vi "Save2DArrayWithColumnNames.vi"(7 "format (%6e)":string="%6e", 8 "error in (no error)":errorcluster, 9 "2D data":dbl[][](array[numeric]), 10 "Column name array":string[](array[string]), 11 "path in":path) -> (0 "error out":errorcluster, 3 "path out":path)   [LabVIEW 2020, in "Initialization.lvlib" / "FileManagement.lvlib"]
uses:
  FileManagement.lvlib
  <vilib>/Utility/error.llb/DialogType.ctl
  <vilib>/Utility/file.llb/Write To Spreadsheet File (DBL).vi
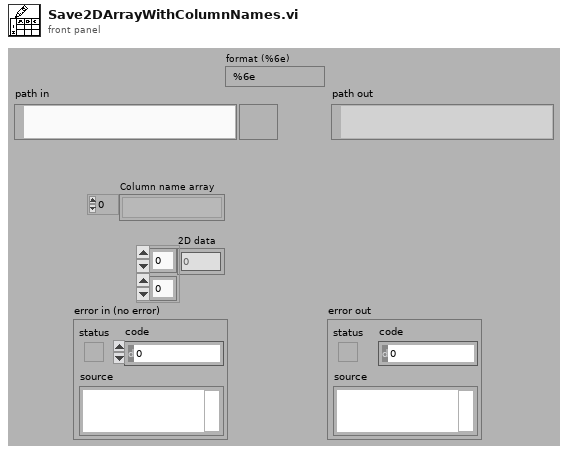
[diagram p1: front panel]
types:
  T1 = enum16{"open", "replace", "create", "open or create", "replace or create", "replace or create with confirmation"}
  T2 = typedef "DialogType.ctl" = u16
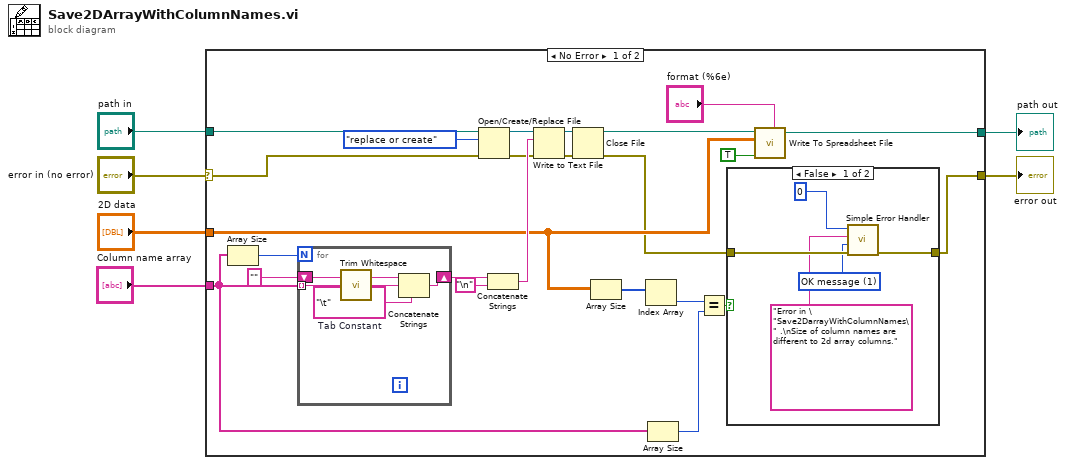
[diagram p0: block diagram]
diagram:
  n1 = case shown="No Error" "error in (no error)" {
    selector: "error in (no error)" -> [w17 w43]
    tunnel: "path in" -> [w16 w42]
    tunnel: "2D data" -> [w15 _]
    tunnel: [w29 w42] -> w5
    tunnel: "Column name array" -> [w14 _]
    tunnel: [w8 w43] -> w4
    frame No Error {
      n2 = Array Size(array=w14) -> (size(s)=w28:i32)
      n3 = for {
        N: w28 -> [_]
        tunnel: w14 -> [w38] mode=indexing
        shift-right: [w41] -> w25
        shift-left: "" -> [w39]
        w40 = "\t"  # Tab Constant
        n4 = call <vilib>:"Trim Whitespace.vi"("string"=w38) -> ("trimmed string"=w37:string)  [unwired: 1 in]
        n5 = Concatenate Strings(w39, w37, w40) -> (w41:string)
      }
      n6 = Open/Create/Replace File(file path (use dialog)=w16, error in=w17, operation (0:open)=T1."replace or create" ("操作(0:open)")) -> (refnum out=w22:refnum<file>, error out=w20:errorcluster)  [unwired: 3 in, 1 out]
      n7 = Concatenate Strings(w25, "\n") -> (w26:string)
      n8 = Write to Text File(file (use dialog)=w22, text=w26, error in=w20) -> (refnum out=w21:refnum<file>, error out=w19:errorcluster)  [unwired: 1 in, 1 out]
      n9 = Close File(refnum=w21, error in=w19) -> (path=w30:path, error out=w9:errorcluster)
      n10 = Array Size(array=w15) -> (size(s)=w13:i32[])
      n11 = Index Array(array=w13) -> (element=w12:i32)  [unwired: 1 in]
      n12 = Array Size(array=w14) -> (size(s)=w11:i32)
      n13 = Equal?(x=w12, y=w11) -> (x = y?=w10:bool)
      n14 = case shown="False" w10 {
        tunnel: w9 -> [w35 w36]
        tunnel: [w34 w36] -> w8
        frame False {
          w32 = T2 1 items=["no dialog", "OK message", "continue or stop message", "OK message + warnings", "continue/stop + warnings"] ("type of dialog (OK msg:1)")
          n15 = call <vilib>:"Simple Error Handler.vi"("error code (no error:0)"=0, "error source (\" \")"="Error in \"Save2DarrayWithColumnNames\" .\nSize of column names are different to 2d array columns." ("error source (\" \")"), "type of dialog (OK msg:1)"=w32, "error in (no error)"=w35) -> ("error out"=w34:errorcluster)  [unwired: 1 in, 4 out]
        }
        frame True {
        }
      }
      n16 = call-poly <vilib>:"Write To Spreadsheet File.vi"("format (%.3f)"="format (%6e)", "append to file? (new file:F)"=TRUE, "2D data"=w15, "file path (dialog if empty)"=w30) -> ("new file path (Not A Path if cancelled)"=w29:path)  [unwired: 4 in]
    }
    frame Error {
    }
  }
  "path out" <- w5
  "error out" <- w4
